vi "Virtual shutter close on live imaging stop.vi"(8 "error in (no error)":errorcluster) -> (0 "error out":errorcluster)   [LabVIEW 2017]
uses:
  Typedefs/Read Write Enum.ctl
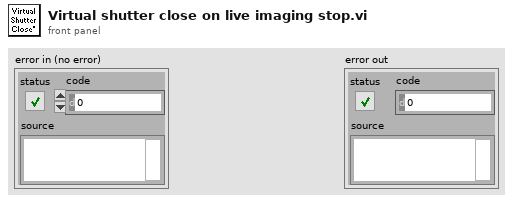
[diagram p1: front panel]
types:
  T1 = typedef "Read Write Enum.ctl" = enum16{"Read", "Write"}
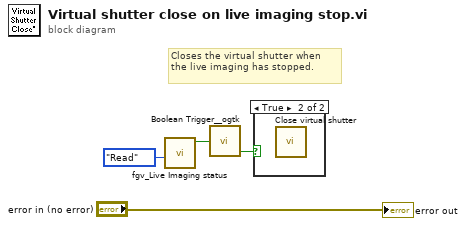
[diagram p0: block diagram]
diagram:
  # "Closes the virtual shutter when the live imaging has stopped."
  n1 = call "fgv_Live Imaging status.vi"("Function"=Read_Write_Enum."Read") -> ("Live Imaging?"=w1:bool)  [unwired: 9 in, 1 out]
  n2 = call <userlib>:"Boolean Trigger__ogtk.vi"("Boolean Input"=w1) -> ("Falling Edge"=w4:bool)  [unwired: 1 in, 1 out]
  n3 = case shown="True" w4 {
    frame False {
    }
    frame True {
      n4 = call "Close virtual shutter.vi"() -> ()  [unwired: 11 in, 1 out]
    }
  }
  "error out" <- "error in (no error)"
